vi "Default Test App Path.vi"() -> (0 "Exe Path":path, 1 "Exe Path With Extention":path)   [LabVIEW 2020, in "serenial.io-ase.test.lvlib"]
uses:
  serenial.io-ase.test.lvlib
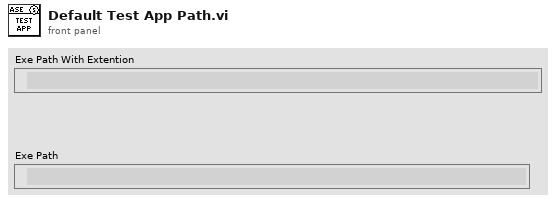
[diagram p1: front panel]
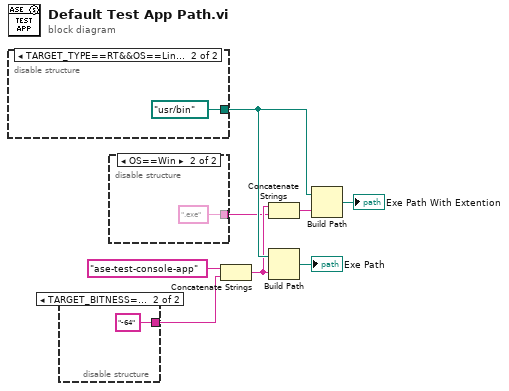
[diagram p0: block diagram]
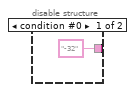
[diagram p3: hidden frame]
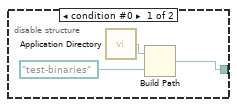
[diagram p4: hidden frame]
diagram:
  n1 = disable-structure shown="TARGET_TYPE==RT&&OS==Linux" {
    disable-tunnel: [w9 path "/usr/bin" ("appended path")] -> w4
    frame condition #0 {
      n2 = call <vilib>:"Application Directory.vi"() -> ("Application Directory"=w10:path)
      n3 = Build Path(base path=w10, name or relative path=path "test-binaries") -> (appended path=w9:path)
    }
    frame condition #1 (active) {
    }
  }
  n4 = disable-structure shown="TARGET_BITNESS==64" {
    disable-tunnel: ["-32" "-64"] -> w7
    frame condition #0 {
    }
    frame condition #1 (active) {
    }
  }
  n5 = disable-structure shown="OS==Win" {
    disable-tunnel: [_ ".exe"] -> w1
    frame condition #0 (active) {
    }
    frame condition #1 {
    }
  }
  n6 = Concatenate Strings("ase-test-console-app", w7) -> (w3:string)
  n7 = Concatenate Strings(w3, w1) -> (w2:string)
  n8 = Build Path(base path=w4, name or relative path=w3) -> (appended path=→"Exe Path":path)
  n9 = Build Path(base path=w4, name or relative path=w2) -> (appended path=→"Exe Path With Extention":path)
